vi "Decompose Cluster - Mixed - Element Type.vi"() -> ()   [LabVIEW 2017, in "Composition.Tests.lvlib"]
uses:
  Composition.Tests.lvlib
  Composition/Composition.lvlib
  <vilib>/Utility/Data Type/NI_Data Type.lvlib
  <vilib>/Utility/Data Type/Type Definitions/Data Type.ctl
  <vilib>/addons/_JKI Toolkits/Caraya/classes/Test/Test.lvclass
  <vilib>/addons/_JKI Toolkits/Caraya/classes/Assert/Assert.lvclass
panel:
  out "error out":errorcluster
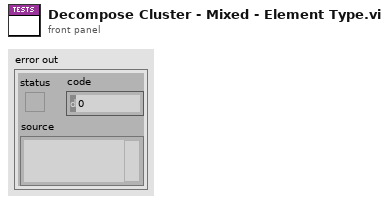
[diagram p1: front panel]
types:
  T1 = typedef "NI_Data Type.lvlib/Data Type.ctl" = enum8{"Invalid Type", "Void", "I8", "I16", "I32", "I64", "U8", "U16", "U32", "U64", "Single Float", "Double Float", "Extended Float", "Single Complex", "Double Complex", "Extended Complex", "Enum U8", "Enum U16", "Enum U32", "Enum U64", "Single Float With Unit", "Double Float With Unit", "Extended Float With Unit", "Single Complex with Unit", "Double Complex with Unit", "Extended Complex with Unit", "Boolean", "String", "Path", "Picture", "Tag", "Array", "Cluster", "Variant", "LV Variant", "Waveform", "Timestamp", "Digital Waveform", "Digital Data", "ExpressData", "Refnum", "External Data", "VI", "Poly VI", "LabVIEW Class Instance", "Fixed Point", "Set Collection", "Map Collection"}
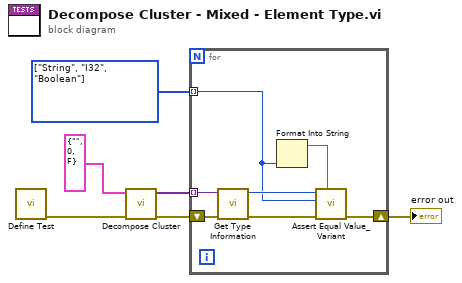
[diagram p0: block diagram]
diagram:
  w3 = T1[] [enum."String", enum."I32", enum."Boolean"] items=["Invalid Type", "Void", "I8", "I16", "I32", "I64", "U8", "U16", "U32", "U64", "Single Float", "Double Float", "Extended Float", "Single Complex", "Double Complex", "Extended Complex", "Enum U8", "Enum U16", "Enum U32", "Enum U64", "Single Float With Unit", "Double Float With Unit", "Extended Float With Unit", "Single Complex with Unit", "Double Complex with Unit", "Extended Complex with Unit", "Boolean", "String", "Path", "Picture", "Tag", "Array", "Cluster", "Variant", "LV Variant", "Waveform", "Timestamp", "Digital Waveform", "Digital Data", "ExpressData", "Refnum", "External Data", "VI", "Poly VI", "LabVIEW Class Instance", "Fixed Point", "Set Collection", "Map Collection"] ("type")
  n1 = call <vilib>:"Define Test.vi"() -> ("error out"=w1:errorcluster)  [unwired: 11 in]
  n2 = call "Decompose Cluster.vi"("error in (no error)"=w1, "Cluster"=cluster{string, i32, bool} {"", 0, FALSE}) -> ("error out"=w5:errorcluster, "Cluster Elements"=w2:variant[])  [unwired: 8 in]
  n3 = for {
    shift-right: [w11] -> w4
    shift-left: w5 -> [w13]
    tunnel: w3 -> [w8] mode=indexing
    tunnel: w2 -> [w10] mode=indexing
    n4 = call <vilib>:"Get Type Information.vi"("error in (no error)"=w13, "variant"=w10) -> ("error out"=w12:errorcluster, "type"=w9:T1)  [unwired: 5 in, 3 out]
    n5 = Format Into String(w8) -> (resulting string=w7:string)  [unwired: 3 in, 1 out]
    n6 = call <vilib>:"Assert Equal Value_Variant.vi"("Label"=w7, "error in (no error)"=w12, "Y"=w8, "X"=w9) -> ("error out"=w11:errorcluster)  [unwired: 7 in]
  }
  "error out" <- w4
